vi "HRM-Stage4-Hardware_simulation_main.vi"(8 "error in (no error)":errorcluster, 11 "Init cluster":T1) -> (0 "error out":errorcluster)   [LabVIEW 2020]
uses:
  initclose/HRM-Stage4-init_cluster.ctl
  initclose/HRM-Stage4-User_events.ctl
panel:
  in  "Aqn?":bool
  in  "stop":bool
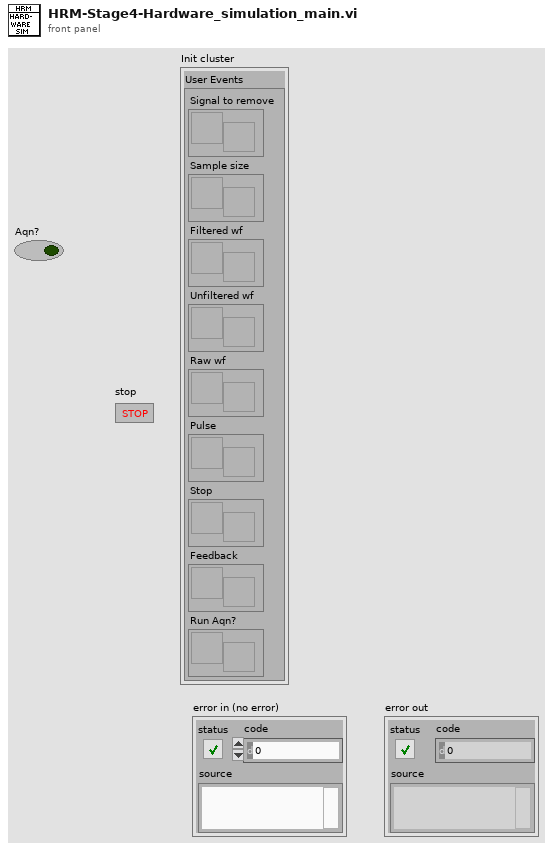
[diagram p1: front panel]
types:
  T1 = typedef "HRM-Stage4-init_cluster.ctl" = cluster{"User Events":T2}
  T2 = typedef "HRM-Stage4-User_events.ctl" = cluster{"Signal to remove":refnum<user-event>, "Sample size":refnum<user-event>, "Filtered wf":refnum<user-event>, "Unfiltered wf":refnum<user-event>, "Raw wf":refnum<user-event>, "Pulse":refnum<user-event>, "Stop":refnum<user-event>, "Feedback":refnum<user-event>, "Run Aqn?":refnum<user-event>}
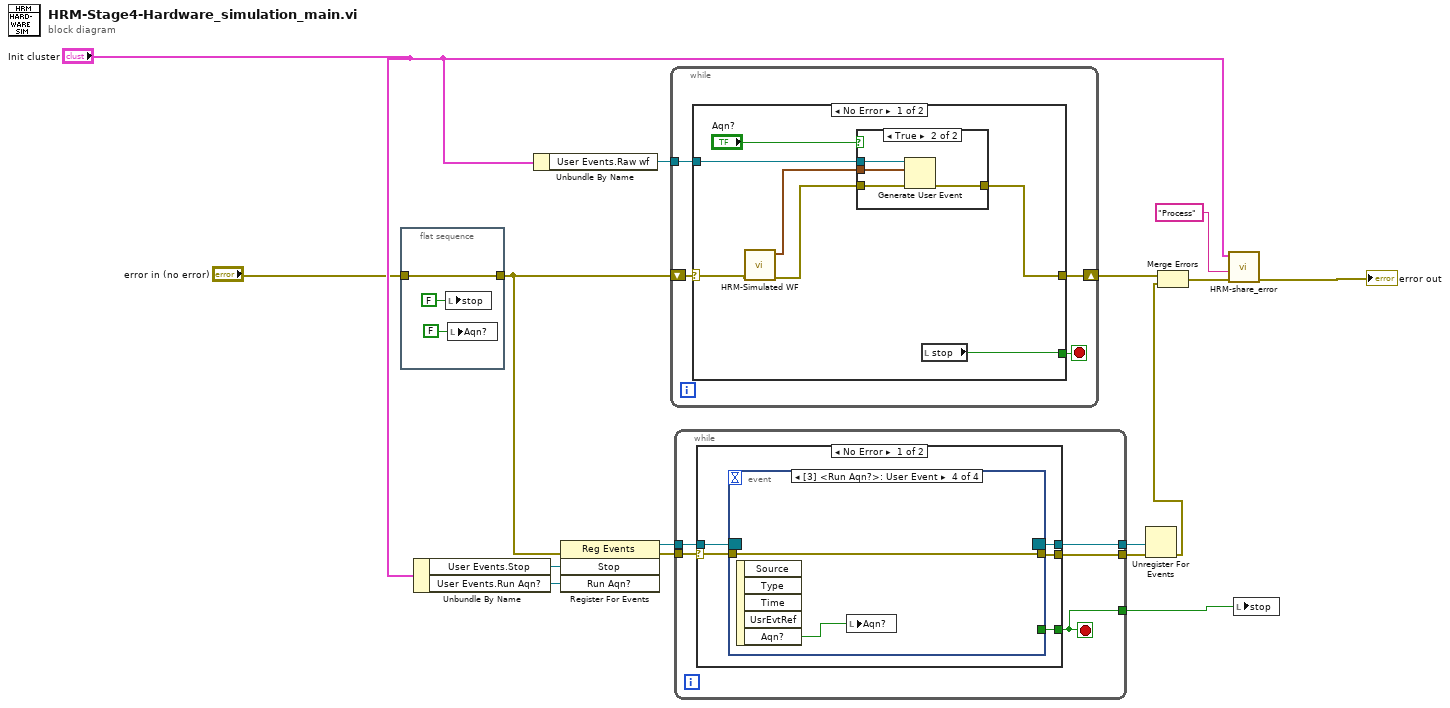
[diagram p0: block diagram]
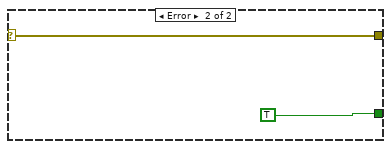
[diagram p3: hidden frame]
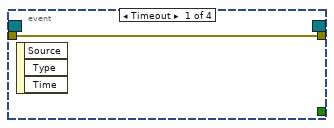
[diagram p4: hidden frame]
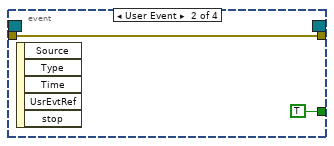
[diagram p5: hidden frame]
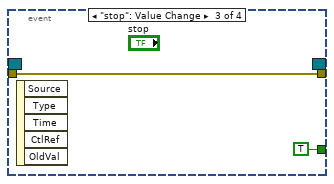
[diagram p6: hidden frame]
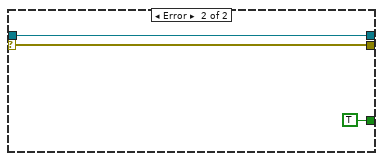
[diagram p7: hidden frame]
diagram:
  n1 = flat-sequence {
    tunnel: "error in (no error)" -> [w19]
    tunnel: [w19] -> w8
    frame #0 {
      n2 = local write "stop"(FALSE ("stop")) -> ()
      n3 = local write "Aqn?"(FALSE ("Aqn?")) -> ()
    }
  }
  n4 = Unbundle By Name("Init cluster") -> ("User Events.Stop"=w12:refnum<user-event>, "User Events.Run Aqn?"=w4:refnum<user-event>)
  n5 = Unbundle By Name("Init cluster") -> ("User Events.Raw wf"=w10:refnum<user-event>)
  n6 = register-events(error in=w8, w12, w4) -> (reference out=w13:refnum<event-registration>, error out=w11:errorcluster)  [unwired: 1 in]
  n7 = while {
    shift-right: [w22] -> w9
    shift-left: w8 -> [w23]
    tunnel: w10 -> [w20]
    stop <- w21 stop-if-true
    n8 = case shown="No Error" w23 {
      selector: w23 -> [w26 w36]
      tunnel: [w30 w36] -> w22
      tunnel: [w28 TRUE ("Stop")] -> w21
      tunnel: w20 -> [w29 _]
      frame No Error {
        n9 = call "HRM-Simulated WF.vi"("error in (no error)"=w26) -> ("error out"=w25:errorcluster, "signal out"=w24:waveform(dbl))  [unwired: 9 in]
        n10 = case shown="True" "Aqn?" {
          tunnel: [w31 w35] -> w30
          tunnel: w29 -> [_ w34]
          tunnel: w25 -> [w31 w33]
          tunnel: w24 -> [_ w32]
          frame False {
          }
          frame True {
            n11 = Generate User Event(user event=w34, event data cluster=w32, error in=w33) -> (error out=w35:errorcluster)  [unwired: 1 in, 1 out]
          }
        }
        n12 = local read "stop"() -> (w28:bool)
      }
      frame Error {
      }
    }
  }
  n13 = while {
    tunnel: w11 -> [w42]
    tunnel: w13 -> [w41]
    tunnel: [w40] -> w14
    tunnel: [w39] -> w15
    tunnel: [w38] -> w7
    stop <- w38 stop-if-true
    n14 = case shown="No Error" w42 {
      selector: w42 -> [w45 w56]
      tunnel: w41 -> [w47 w55]
      tunnel: [w46 TRUE] -> w38
      tunnel: [w44 w56] -> w39
      tunnel: [w43 w55] -> w40
      frame No Error {
        n15 = event shown="[3] <Run Aqn?>: User Event" {
          selector: w47 -> [_ _ _ _]
          dyn-events: [_ _ _ _] -> w43
          timeout: _ -> [_ _ _ _]
          tunnel: [_ TRUE TRUE _] -> w46
          tunnel: w45 -> [w48 w49 w52 w54]
          tunnel: [w48 w49 w52 w54] -> w44
          event Timeout {
            n16 = event-data() -> ()  [unwired: 1 in, 3 out]
          }
          event User Event {
            n17 = event-data() -> ()  [unwired: 1 in, 5 out]
          }
          event "stop": Value Change {
            n18 = event-data() -> ()  [unwired: 1 in, 5 out]
          }
          event User Event {
            n19 = event-data() -> ("Aqn?"=w53:bool)  [unwired: 1 in, 4 out]
            n20 = local write "Aqn?"(w53) -> ()
          }
        }
      }
      frame Error {
      }
    }
  }
  n21 = Unregister For Events(event registration refnum=w14, error in=w15) -> (error out=w16:errorcluster)
  n22 = Merge Errors(w9, w16) -> (w5:errorcluster)
  n23 = call "HRM-share_error.vi"("error in (no error)"=w5, "module name"="Process", "Init cluster"="Init cluster") -> ("error out"=→"error out":errorcluster)  [unwired: 8 in]
  n24 = local write "stop"(w7) -> ()
